vi "Problem1.7.vi"() -> ()   [LabVIEW 2019]
panel:
  in  "Copy New Last Name":bool=TRUE
  in  "New Last Name":string
  out "Output Cluster":cluster{"First Name":string, "Last Name":string}
  in  "Input Cluster":cluster{"First Name":string, "Last Name":string}={"First Name"="Jeff", "Last Name"="Brusoe\nBrusoe"}
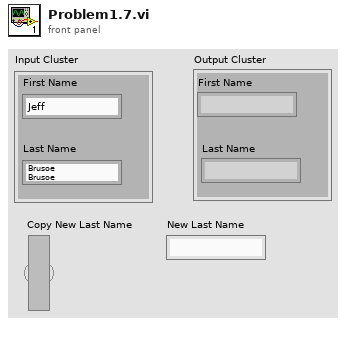
[diagram p1: front panel]
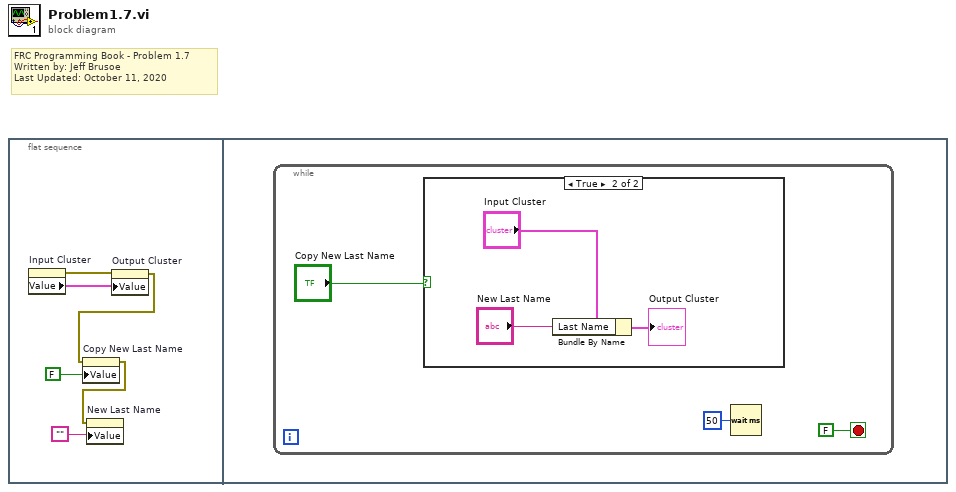
[diagram p0: block diagram]
diagram:
  # "FRC Programming Book - Problem 1.7\nWritten by: Jeff Brusoe\nLast Updated: October 11, 2020"
  n1 = flat-sequence {
    frame #0 {
      n2 = property on="Input Cluster" class="Clust (strict)"() -> (error out=w4:errorcluster, "Value"=w6:cluster{"First Name":string, "Last Name":string})  [unwired: 2 in, 1 out]
      n3 = property on="Output Cluster" class="Clust (strict)"(error in=w4, "Value"=w6) -> (error out=w3:errorcluster)  [unwired: 1 in, 1 out]
      n4 = property on="Copy New Last Name" class="Bool (strict)"(error in=w3, "Value"=FALSE) -> (error out=w2:errorcluster)  [unwired: 1 in, 1 out]
      n5 = property on="New Last Name" class="Str"(error in=w2, "Value"="") -> ()  [unwired: 1 in, 2 out]
    }
    frame #1 {
      n6 = while {
        stop <- FALSE stop-if-true
        n7 = case shown="True" "Copy New Last Name" {
          frame False {
          }
          frame True {
            n8 = Bundle By Name(cluster="Input Cluster", "Last Name"="New Last Name") -> (→"Output Cluster":cluster{"First Name":string, "Last Name":string})
          }
        }
        n9 = Wait (ms)(milliseconds to wait=u32 50) -> ()  [unwired: 1 out]
      }
    }
  }
